vi "Robot Global Data.vi"() -> ()   [LabVIEW 2015]
doc: "This global VI can contain as many global variables as you need. Place a control on the panel, give it a good name. To read or write to it from a VI, drag the icon to the diagram of that VI. You can also drag from the project. Click on the node to change which global you access. You shouldn't have multiple locations writing to a global or it will cause a race-condition."
uses:
  <vilib>/Rock Robotics/WPI/Camera/WPI_CameraImageSize.ctl
  <vilib>/Rock Robotics/WPI/DriverStation/WPI_DriverStationRobotMode2.ctl
panel:
  in  "Current Target Location":cluster{"X":dbl, "Y":dbl}
  in  "Current Image Size":cluster{"X":i32, "Y":i32}
  in  "Ball Intake Start Time":u32
  in  "Gyro Angles":T1
  in  "Drive Task Async Enabled":bool
  in  "Drive Task Mode":enum16{"Synchronous", "Asynchronous"}(ring)
  in  "Drive Task Parameters":T2
  in  "Ball Shooter Async Enabled":bool
  in  "Ball Shooter Task Mode":enum16{"Synchronous", "Asynchronous"}(ring)
  in  "Ball Shooter Task Parameters":T3
  in  "Simulated":bool
  in  "Robot Mode":T4
  in  "image size":T5=enum."320x240"
  in  "Enable Vision":bool
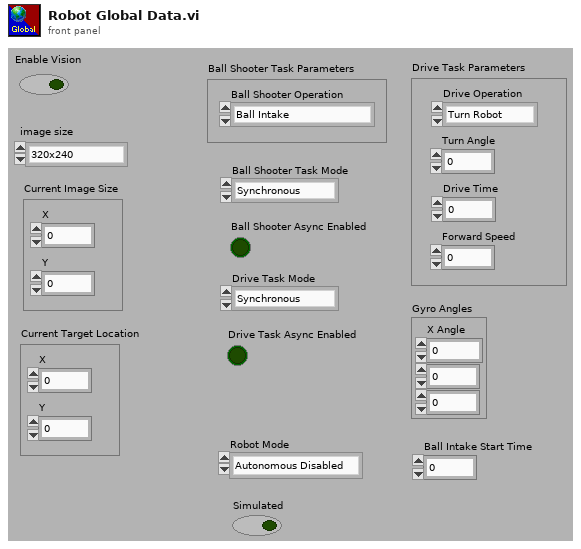
[diagram p1: front panel]
types:
  T1 = cluster{"X Angle":dbl, "Y Angle":dbl, "Z Angle":dbl}
  T2 = cluster{"Turn Angle":dbl, "Drive Time":dbl, "Forward Speed":dbl, "Drive Operation":enum16{"Turn Robot", "Drive Straight for Time", "Drive to Obstacle Start"}}
  T3 = cluster{"Ball Shooter Operation":enum16{"Ball Intake", "Fire Ball Shooter", "Aim Ball Shooter"}}
  T4 = typedef "WPI_DriverStationRobotMode2.ctl" = enum16{"Autonomous Disabled", "Autonomous Enabled", "Teleop Disabled", "Teleop Enabled", "Disconnected", "Finish", "Test Disabled", "Test Enabled", "Emergency Stopped"}
  T5 = typedef "WPI_CameraImageSize.ctl" = enum16{"640x480", "320x240", "160x120", "Custom"}
diagram:
